vi "DataTypes Error Core.vi"(8 "error in (no error)":errorcluster, 10 "String to Append":string, 11 "Error":T1) -> (0 "error out":errorcluster)   [LabVIEW 2021, in "DataTypes_CIF_U.lvlib"]
uses:
  DataTypes_CIF_U.lvlib
  Typedef/Errors.ctl
  Errors/Errors_CIF_U.lvlib
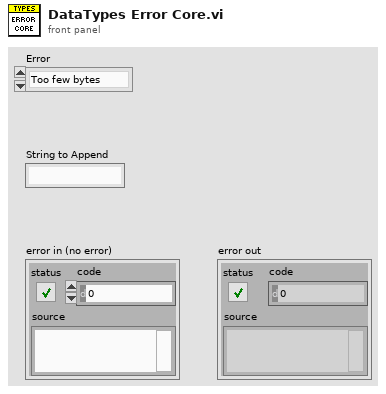
[diagram p1: front panel]
types:
  T1 = typedef "DataTypes_CIF_U.lvlib/Errors.ctl" = enum16{"Too few bytes", "Unsupported Type", "Invalid GUID", "Error Parsing JSON"}
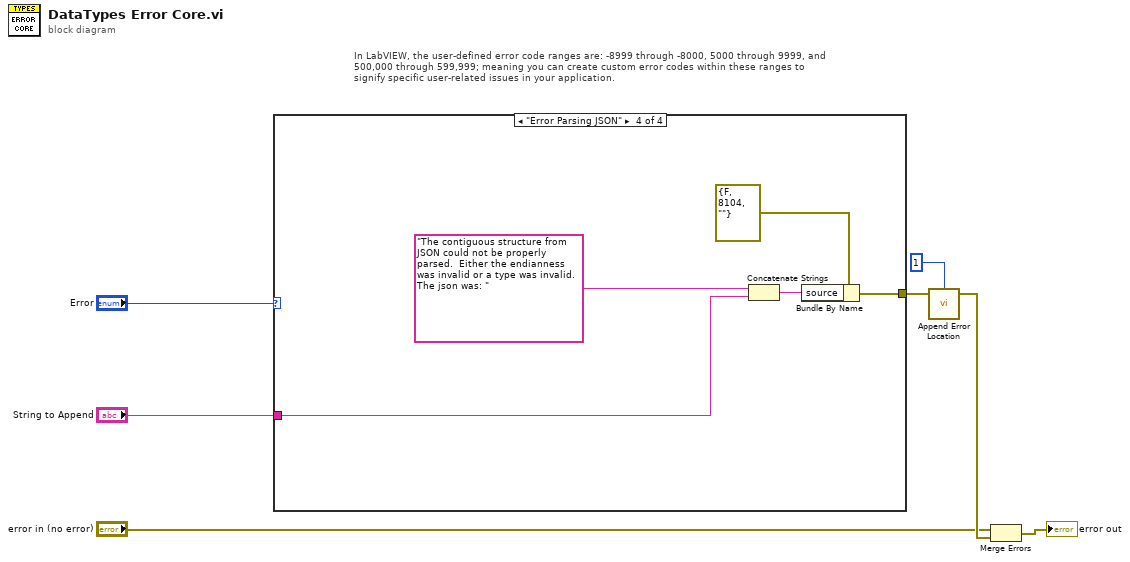
[diagram p0: block diagram]
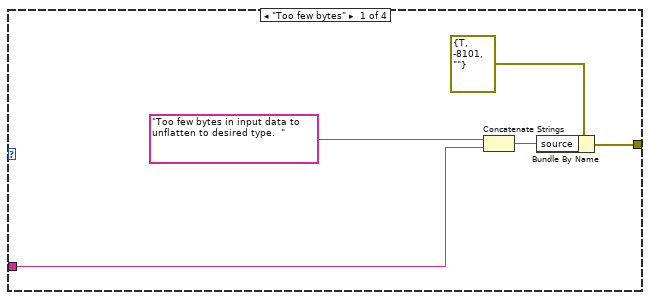
[diagram p2: hidden frame]
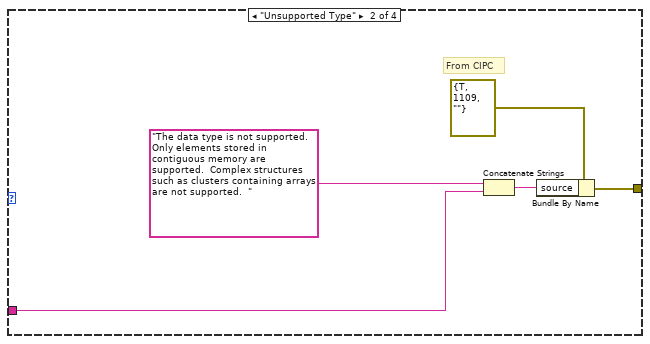
[diagram p3: hidden frame]
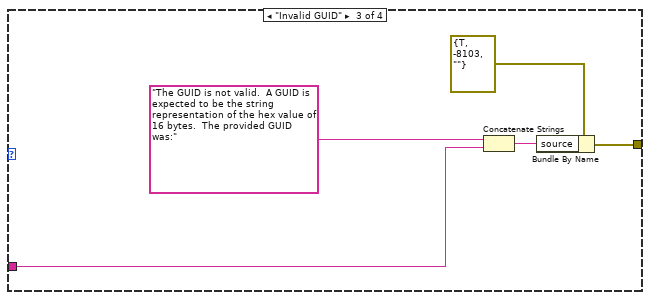
[diagram p4: hidden frame]
diagram:
  # "In LabVIEW, the user-defined error code ranges are: -8999 through -8000, 5000 through 9999, and 500,000 through 599,999; meaning you can create custom error codes within these ranges to signify specific user-related issues in your application."
  n1 = case shown="\"Error Parsing JSON\"" "Error" {
    tunnel: "String to Append" -> [w9 w14 w19 w24]
    tunnel: [w11 w16 w21 w26] -> w6
    frame "Too few bytes" {
      n2 = Concatenate Strings("Too few bytes in input data to unflatten to desired type.  " ("source"), w9) -> (w8:string)
      n3 = Bundle By Name(cluster=errorcluster {"status"=TRUE, "code"=-8101, "source"=""} ("Invalid ID"), "source"=w8) -> (w11:errorcluster)
    }
    frame "Unsupported Type" {
      # "From CIPC"
      n4 = Concatenate Strings("The data type is not supported.  Only elements stored in contiguous memory are supported.  Complex structures such as clusters containing arrays are not supported.  " ("source"), w14) -> (w13:string)
      n5 = Bundle By Name(cluster=errorcluster {"status"=TRUE, "code"=1109, "source"=""} ("Invalid ID"), "source"=w13) -> (w16:errorcluster)
    }
    frame "Invalid GUID" {
      n6 = Concatenate Strings("The GUID is not valid.  A GUID is expected to be the string representation of the hex value of 16 bytes.  The provided GUID was:" ("source"), w19) -> (w18:string)
      n7 = Bundle By Name(cluster=errorcluster {"status"=TRUE, "code"=-8103, "source"=""} ("Invalid ID"), "source"=w18) -> (w21:errorcluster)
    }
    frame "Error Parsing JSON" {
      n8 = Concatenate Strings("The contiguous structure from JSON could not be properly parsed.  Either the endianness was invalid or a type was invalid.  The json was: " ("source"), w24) -> (w23:string)
      n9 = Bundle By Name(cluster=errorcluster {"status"=FALSE, "code"=8104, "source"=""} ("Invalid ID"), "source"=w23) -> (w26:errorcluster)
    }
  }
  n10 = call "Append Error Location.vi"("error in (no error)"=w6, "Chain Depth"=1) -> ("error out"=w7:errorcluster)  [unwired: 3 in]
  n11 = Merge Errors("error in (no error)", w7) -> (→"error out":errorcluster)
